vi "Logger_Core.vi"(8 "error in (no error)":errorcluster caption="错误输入（无错误）", 11 "Logger 输入":refnum<class "Logger.lvclass">) -> (0 "error out":errorcluster caption="错误输出", 3 "Logger 输出":refnum<class "Logger.lvclass">)   [LabVIEW 2019, in "Logger.lvclass"]
uses:
  <userlib>/Logger/Logger.lvclass
  <userlib>/Logger/Logger.lvclass/Logger.ctl
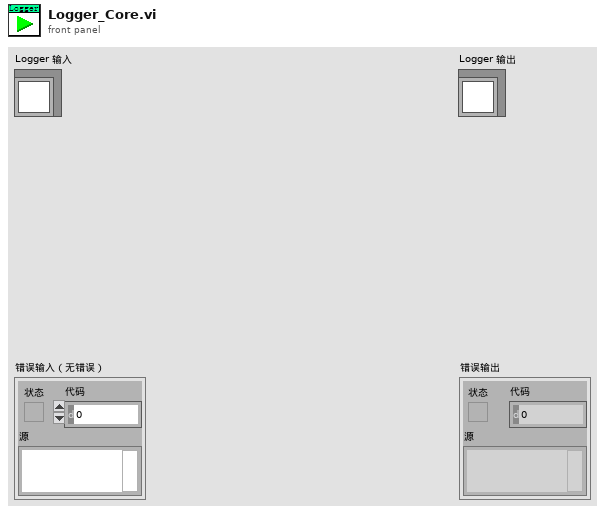
[diagram p1: front panel]
types:
  T1 = typedef "Logger.lvclass/LoggerMessage.ctl" = cluster{"LoggerKind":enum16{"软件上传日志", "软件其他日志", "软件错误日志", "软件监控日志"}, "LoggerMessage":string, "LoggerCode":i32, "LoggerCallChain":string, "LoggerTime":string}
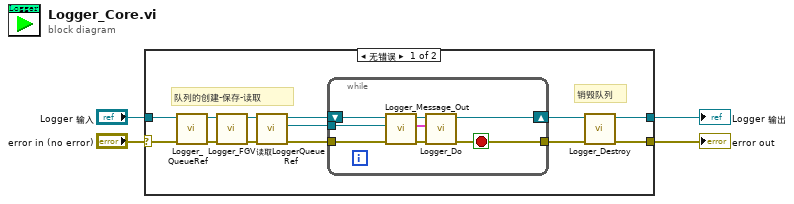
[diagram p0: block diagram]
diagram:
  n1 = case shown="无错误" "error in (no error)" {
    selector: "error in (no error)" -> [w7 w27]
    tunnel: [w11 w27] -> w3
    tunnel: [w13 w26] -> w1
    tunnel: "Logger 输入" -> [w8 w26]
    frame No Error {
      # "销毁队列"
      # "队列的创建-保存-读取"
      n2 = call <userlib>:"Logger_QueueRef.vi"("error in (no error)"=w7, "Logger 输入"=w8) -> ("error out"=w9:errorcluster, "Logger 输出"=w10:refnum<class "Logger.lvclass">)  [unwired: 8 in]
      n3 = call <userlib>:"Logger_FGV.vi"("error in (no error)"=w9, "Logger 输入"=w10) -> ("error out"=w5:errorcluster, "Logger 输出"=w6:refnum<class "Logger.lvclass">)  [unwired: 8 in]
      n4 = call "读取LoggerQueueRef.vi"("error in (no error)"=w5, "Logger输入"=w6) -> ("error out"=w17:errorcluster, "LoggerQueueRef"=w16:refnum<queue>, "Logger输出"=w15:refnum<class "Logger.lvclass">)  [unwired: 7 in]
      n5 = while {
        tunnel: w17 -> [w23]
        tunnel: [w18] -> w12
        shift-right: [w19] -> w14
        shift-left: w15 -> [w25]
        tunnel: w16 -> [w24]
        stop <- w18 stop-if-true
        n6 = call <userlib>:"Logger_Message_Out.vi"("error in (no error)"=w23, "LoggerQueueRef"=w24, "Logger 输入"=w25) -> ("error out"=w20:errorcluster, "Message"=w21:T1, "Logger 输出"=w22:refnum<class "Logger.lvclass">)  [unwired: 6 in]
        n7 = call <userlib>:"Logger_Do.vi"("error in (no error)"=w20, "Message"=w21, "Logger 输入"=w22) -> ("error out"=w18:errorcluster, "Logger 输出"=w19:refnum<class "Logger.lvclass">)  [unwired: 7 in]
      }
      n8 = call <userlib>:"Logger_Destroy.vi"("error in (no error)"=w12, "Logger 输入"=w14) -> ("error out"=w11:errorcluster, "Logger 输出"=w13:refnum<class "Logger.lvclass">)  [unwired: 8 in]
    }
    frame Error {
    }
  }
  "error out" <- w3
  "Logger 输出" <- w1
